vi "Image UDP Broadcast GUID Lookup.vi"() -> ()   [LabVIEW 2012, in "Image UDP Broadcast Custom Device.lvlib"]
doc: "Use this Global VI to access the GUIDs assigned to the page resources of the Custom Device."
uses:
  Image UDP Broadcast Custom Device.lvlib
panel:
  in  "Error Status":string="1a3d95e5-e85d-492e-bfbe-a8a7a366c366"
  in  "Valid Bytes per Packet":string="d3b435dc-7be6-45d2-8de9-02e428f39193"
  in  "Broadcast Page":string="fe5ed426-67fa-4d12-8664-845fa0bcf859"
  in  "Broadcast Status":string="cae686a1-7c8e-428f-b7cd-999c0bc074d0"
  in  "Custom Device":string="b05a5688-3b16-44fb-bff1-faa0fcd6f436"
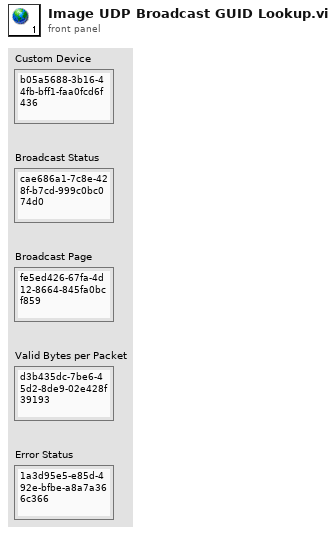
[diagram p1: front panel]
diagram:
